vi "OAT Polar Draw Plot.vi"(6 "channel settings":T1 {"probe angle [deg]" max=360 step=1; "shaft rotating direction" items=["CCW", "CW"]}, 7 "polar settings":T2={"polar attributes"={"maximum"=2.0, "minimum"=0.0, "clip to min"=FALSE, "log"=FALSE, "grid color"=3381657, "plot color"=16711680, "fmt and prec"={"format"=enum."Decimal", "precision"=2}, "visible section"=4}, "desired font"=enum."Application Font", "user-specified font"={"Font Name:"="", "Size"=0, "Strikeout?"=FALSE, "Italic?"=FALSE, "Underline?"=FALSE, "Outline?"=FALSE, "Shadow?"=FALSE, "Bold?"=FALSE}} {"polar attributes"."minimum" format="%.2f"; "polar attributes"."maximum" format="%.2f"}, 8 "top left point(0, 0)":cluster{"x":i16, "y":i16}, 9 "dimensions (w,h)":cluster{"width":i16, "height":i16}, 10 "data array [mag, phase (deg)]":cluster{"magnitude":dbl, "phase":dbl}[](array[cluster]) {"phase" format="%.2f"; "magnitude" format="%.2f"}, 11 "picture":picture) -> (1 "grid measurements":T3 {"end angle" format="%.2f"; "start angle" format="%.2f"; "scale factors"."b" format="%.2f"; "scale factors"."a" format="%.2f"}, 3 "new picture":picture)   [LabVIEW 2017]
doc: "Takes a picture and polar data and appends a picture that represents a polar graph of the data."
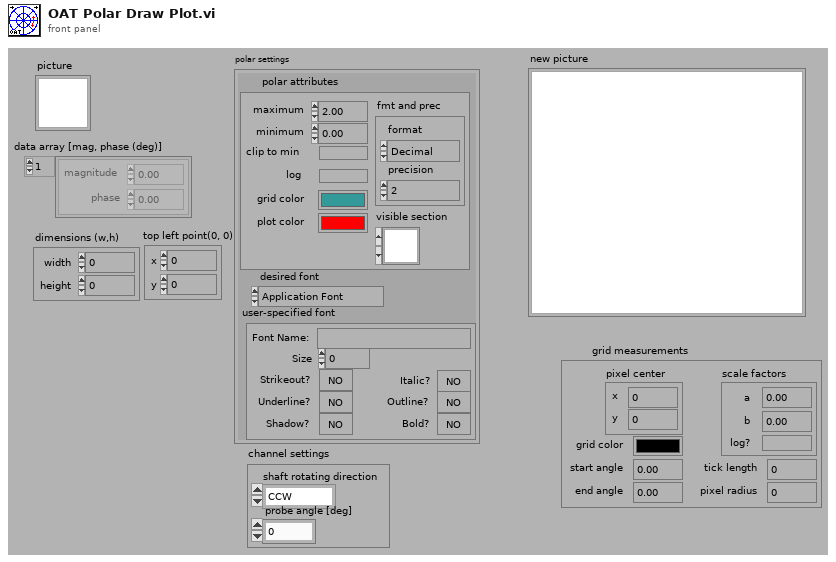
[diagram p1: front panel]
types:
  T1 = cluster{"shaft rotating direction":u16, "probe angle [deg]":u16}
  T2 = cluster{"polar attributes":cluster{"maximum":dbl, "minimum":dbl, "clip to min":bool, "log":bool, "grid color":u32, "plot color":u32, "fmt and prec":cluster{"format":enum8{"Decimal", "Scientific", "Engineering", "Binary", "Octal", "Hex"}, "precision":u8}, "visible section":u16}, "desired font":enum16{"User-specified Font", "Application Font", "System Font", "Dialog Font"}, "user-specified font":cluster{"Font Name:":string, "Size":i16, "Strikeout?":bool, "Italic?":bool, "Underline?":bool, "Outline?":bool, "Shadow?":bool, "Bold?":bool}}
  T3 = cluster{"pixel center":cluster{"x":i16, "y":i16}, "scale factors":cluster{"a":dbl, "b":dbl, "log?":bool}, "grid color":u32, "start angle":dbl, "end angle":dbl, "tick length":i16, "pixel radius":i32}
  T4 = cluster{"maximum":dbl, "minimum":dbl, "clip to min":bool, "log":bool, "grid color":u32, "plot color":u32, "fmt and prec":cluster{"format":enum8{"Decimal", "Scientific", "Engineering", "Binary", "Octal", "Hex"}, "precision":u8}, "visible section":u16}
  T5 = enum16{"User-specified Font", "Application Font", "System Font", "Dialog Font"}
  T6 = cluster{"Font Name:":string, "Size":i16, "Strikeout?":bool, "Italic?":bool, "Underline?":bool, "Outline?":bool, "Shadow?":bool, "Bold?":bool}
  T7 = cluster{"left":i16, "top":i16, "right":i16, "bottom":i16}
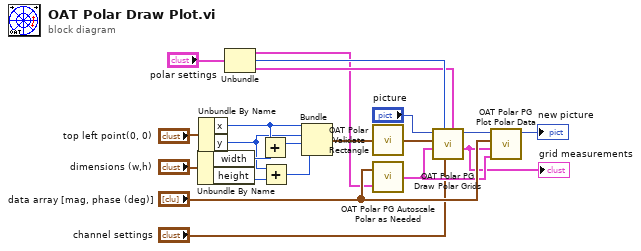
[diagram p0: block diagram]
diagram:
  n1 = Unbundle By Name("dimensions (w,h)") -> ("width"=w12:i16, "height"=w11:i16)
  n2 = Unbundle By Name("top left point(0, 0)") -> ("x"=w10:i16, "y"=w9:i16)
  n3 = Unbundle("polar settings") -> ("polar attributes"=w2:T4, "desired font"=w4:T5, "user-specified font"=w3:T6)
  n4 = Add(x=w10, y=w12) -> (x+y=w8:i16)
  n5 = Add(x=w9, y=w11) -> (x+y=w7:i16)
  n6 = Bundle("x"=w10, "y"=w9, w8, w7) -> (w6:cluster{"x":i16, "y":i16, i16, i16})  [unwired: 1 in]
  n7 = call <vilib>:"OAT Polar Validate Rectangle.vi"("rect"=w6) -> ("valid rect"=w15:T7)
  n8 = call <vilib>:"OAT Polar PG Autoscale Polar as Needed.vi"("polar attributes"=w2, "data"="data array [mag, phase (deg)]") -> ("polar attributes"=w17:T4)
  n9 = call <vilib>:"OAT Polar PG Draw Polar Grids.vi"("[user-specified font]"=w3, "channel settings"="channel settings", "desired font(Application)"=w4, "polar attributes"=w17, "rect"=w15, "picture"="picture") -> ("grid measurements"=w16:T3, "new picture"=w18:picture)  [unwired: 4 in]
  "grid measurements" <- w16
  n10 = call <vilib>:"OAT Polar PG Plot Polar Data.vi"("polar attributes"=w17, "grid measurements"=w16, "polar data"="data array [mag, phase (deg)]", "picture"=w18) -> ("new picture"=→"new picture":picture)  [unwired: 3 in]
